vi "Battery First Match.vi"(7 "Safety Init":bool, 8 "Error In":errorcluster, 9 "PC Data":T1 {"Alarms 2" format="%016b"; "Faults 2" format="%016b"; "Alarms 1" format="%016b"; "Faults 1" format="%016b"; "Contactor FB" format="%.0b"; "DC Voltage SP" format="%2.1f"; "Clear Faults SP" format="%.0b"; "Neutral Current" format="%2.1f"; "AC Current - L2" format="%2.1f"; "AC Voltage - L2" format="%2.1f"; "Temperature" format="%2.1f"; "DC Voltage" format="%2.1f"; "AC Current SP" format="%2.1f"; "AC Voltage SP" format="%2.1f"; "Frequency SP" format="%2.1f"; "AC Frequency" format="%2.1f"; "AC Current - L1" format="%2.1f"; "AC Voltage- L1" format="%2.1f"}, 10 "String Index":i32, 11 "ES String Data":T3) -> (0 "Error Out":errorcluster, 1 "Contactor Closed":bool=TRUE, 2 "ES ON Array":bool[](array[boolean]), 3 "Close Command Sent":bool=TRUE, 5 "DC Link Command":sgl)   [LabVIEW 2014]
uses:
  Controls/ES String Array.ctl
  Controls/ES String Data.ctl
  Controls/PC Data.ctl
  Controls/MicroZed Config Op Mode.ctl
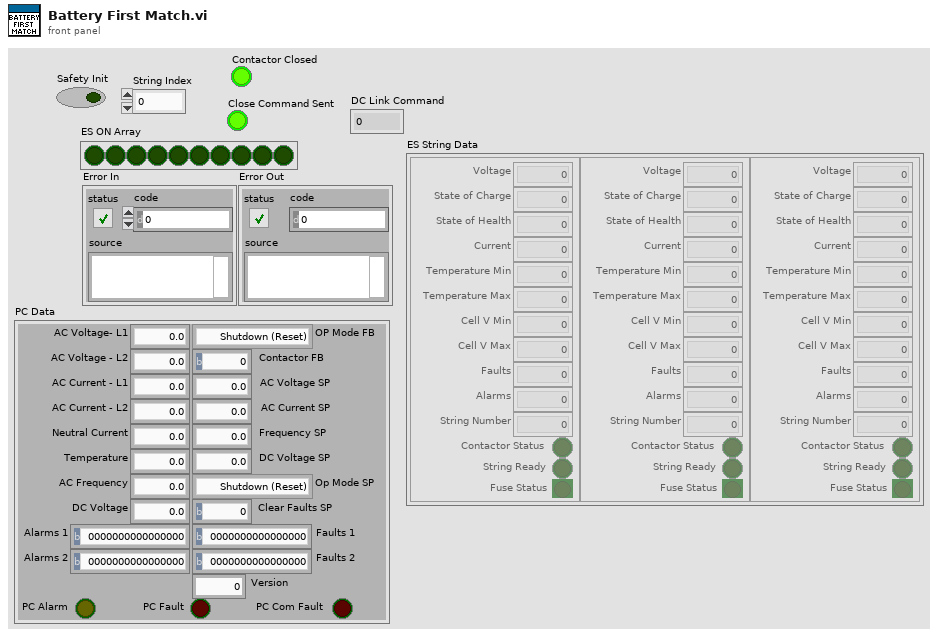
[diagram p1: front panel]
types:
  T1 = typedef "PC Data.ctl" = cluster{"AC Voltage- L1":dbl, "AC Voltage - L2":dbl, "AC Current - L1":dbl, "AC Current - L2":dbl, "Neutral Current":dbl, "Temperature":dbl, "AC Frequency":dbl, "DC Voltage":dbl, "AC Voltage SP":dbl, "AC Current SP":dbl, "Frequency SP":dbl, "Op Mode SP":T2, "Clear Faults SP":u16, "PC Com Fault":bool, "PC Fault":bool, "DC Voltage SP":dbl, "OP Mode FB":T2, "Contactor FB":u16, "Faults 1":u16, "Alarms 1":u16, "Faults 2":u16, "Alarms 2":u16, "PC Alarm":bool, "Version":u16}
  T2 = typedef "MicroZed Config Op Mode.ctl" = enum16{"Shutdown (Reset)", "Startup", "Idle", "Voltage Mode", "Current Mode", "Fault", "OL Voltage (Debug)", "No Data"}
  T3 = typedef "ES String Array.ctl" = T4[]
  T4 = typedef "ES String Data.ctl" = cluster{"Voltage":sgl, "State of Charge":sgl, "Current":sgl, "Temperature Min":i16, "Temperature Max":i16, "Faults":u16, "Alarms":u16, "String Number":u16, "Contactor Status":bool, "String Ready":bool, "Fuse Status":bool, "Cell V Max":dbl, "Cell V Min":dbl, "State of Health":sgl}
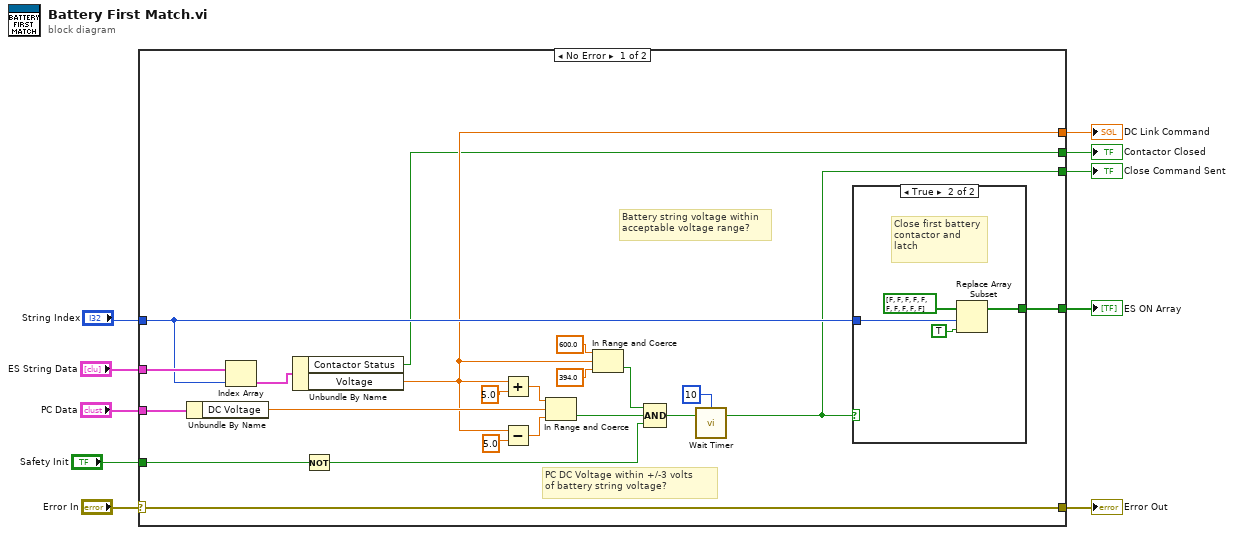
[diagram p0: block diagram]
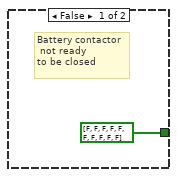
[diagram p2: hidden frame]
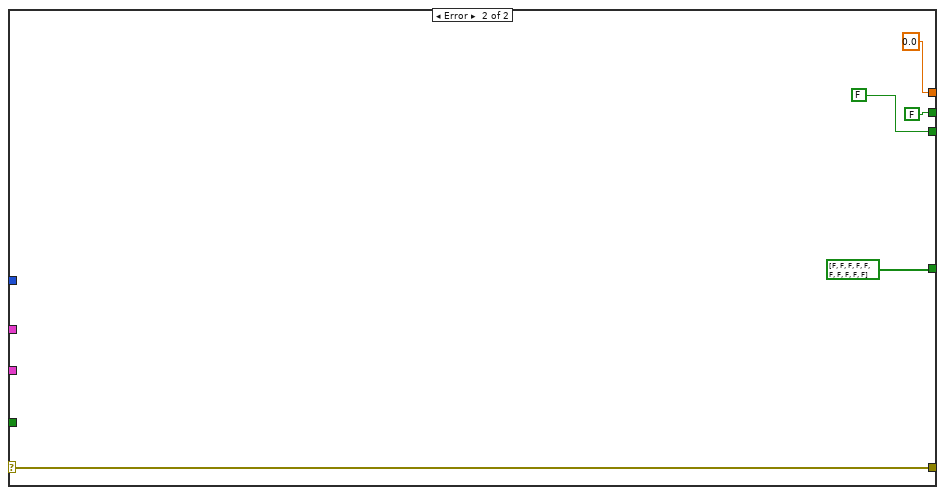
[diagram p3: hidden frame]
diagram:
  n1 = case shown="No Error" "Error In" {
    selector: "Error In" -> [w32 w42]
    tunnel: [w32 w42] -> w9
    tunnel: "ES String Data" -> [w30 _]
    tunnel: "PC Data" -> [w31 _]
    tunnel: [w28 bool[] [FALSE, FALSE, FALSE, FALSE, FALSE, FALSE, FALSE, FALSE, FALSE, FALSE] ("ES ON Array")] -> w6
    tunnel: [w13 FALSE] -> w5
    tunnel: [w15 sgl 0.0 ("Voltage")] -> w4
    tunnel: "String Index" -> [w18 _]
    tunnel: "Safety Init" -> [w14 _]
    tunnel: [w12 FALSE ("Contactor Status")] -> w1
    frame No Error {
      # "Battery string voltage within\nacceptable voltage range?"
      # "PC DC Voltage within +/-3 volts \nof battery string voltage?"
      n2 = Unbundle By Name(w31) -> ("DC Voltage"=w27:dbl)
      n3 = Index Array(array=w30, index=w18) -> (element=w29:T4)
      n4 = Unbundle By Name(w29) -> ("Contactor Status"=w12:bool, "Voltage"=w15:sgl)
      n5 = Not(x=w14) -> (.not. x?=w11:bool)
      n6 = Add(x=w15, y=5.0) -> (x+y=w23:dbl)
      n7 = Subtract(x=w15, y=5.0) -> (x-y=w24:dbl)
      n8 = In Range and Coerce(upper limit=w23, x=w27, lower limit=w24) -> (In Range?=w22:bool)  [unwired: 1 out]
      n9 = In Range and Coerce(upper limit=600.0, x=w15, lower limit=394.0) -> (In Range?=w19:bool)  [unwired: 1 out]
      n10 = Compound Arithmetic op=AND(w19, w22, w11) -> (w17:bool)
      n11 = call "Wait Timer.vi"("Boolean In"=w17, "Timer"=u32 10) -> ("Boolean Out"=w13:bool)  [unwired: 3 in]
      n12 = case shown="True" w13 {
        tunnel: w18 -> [_ w35]
        tunnel: [bool[] [FALSE, FALSE, FALSE, FALSE, FALSE, FALSE, FALSE, FALSE, FALSE, FALSE] ("ES ON Array") w34] -> w28
        frame False {
          # "Battery contactor\n not ready\nto be closed"
        }
        frame True {
          # "Close first battery\ncontactor and\nlatch"
          n13 = Replace Array Subset(array=bool[] [FALSE, FALSE, FALSE, FALSE, FALSE, FALSE, FALSE, FALSE, FALSE, FALSE] ("ES ON Array"), new element=TRUE ("new element/subarray"), index=w35) -> (w34:bool[])
        }
      }
    }
    frame Error {
    }
  }
  "ES ON Array" <- w6
  "Error Out" <- w9
  "Close Command Sent" <- w5
  "DC Link Command" <- w4
  "Contactor Closed" <- w1
